vi "min output.vi"(10 "deadband width":dbl, 11 "motor input":dbl) -> (3 "motor output":dbl)   [LabVIEW 2014]
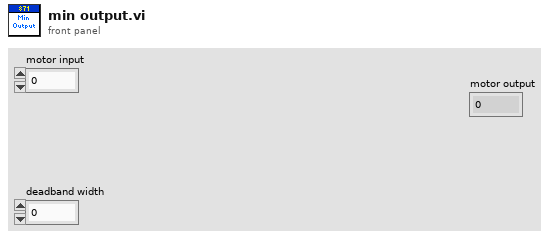
[diagram p1: front panel]
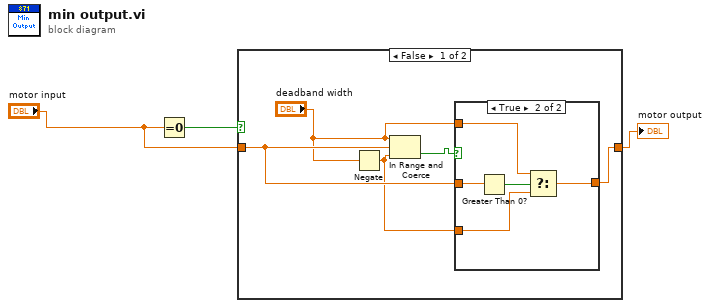
[diagram p0: block diagram]
diagram:
  n1 = Equal To 0?(x="motor input") -> (x = 0?=w3:bool)
  n2 = case shown="False" w3 {
    tunnel: "motor input" -> [w7 w15]
    tunnel: [w6 w15] -> w1
    frame False {
      n3 = Negate(x="deadband width") -> (-x=w4:dbl)
      n4 = In Range and Coerce(upper limit="deadband width", x=w7, lower limit=w4) -> (In Range?=w8:bool)  [unwired: 1 out]
      n5 = case shown="True" w8 {
        tunnel: w7 -> [w9 w14]
        tunnel: [w9 w12] -> w6
        tunnel: "deadband width" -> [_ w11]
        tunnel: w4 -> [_ w10]
        frame False {
        }
        frame True {
          n6 = Greater Than 0?(x=w14) -> (x > 0?=w13:bool)
          n7 = Select(t=w11, s=w13, f=w10) -> (s? t:f=w12:dbl)
        }
      }
    }
    frame True {
    }
  }
  "motor output" <- w1
